vi "Main.vi"() -> ()   [LabVIEW 2019]
uses:
  <vilib>/Platform/TimedLoop/XDataNode/timing_clust.ctl
  <vilib>/Platform/TimedLoop/XDataNode/nitl_modes.ctl
  <vilib>/Platform/TimedLoop/XDataNode/wakeup.ctl
  <vilib>/myRIO/Instrument Drivers/Onboard IO/DIO/typedefs/DIO Reference.ctl
  <vilib>/myRIO/Common/Instrument Driver Framework/Utilities/typedefs/myRIO Generic Hardware Reference.ctl
  <vilib>/myRIO/Common/Instrument Driver Framework/Utilities/typedefs/Hardware Version Enum.ctl
  <vilib>/myRIO/Common/Instrument Driver Framework/Utilities/typedefs/myRIO v1.0 Reference.ctl
  <vilib>/myRIO/Common/Instrument Driver Framework/Utilities/typedefs/Generic FPGA Reference.ctl
  <vilib>/myRIO/Common/Instrument Driver Framework/myRIO v1.0/DIO/typedefs/DIO Channels List.ctl
  <vilib>/myRIO/Common/Instrument Driver Framework/myRIO v1.0/DIO/typedefs/DIO Channels Enum.ctl
  <vilib>/userDefined/High Color/nirio_resource_hc.ctl
  <vilib>/myRIO/Instrument Drivers/Onboard Devices/Accelerometer/typedefs/Accelerometer Reference.ctl
  <vilib>/myRIO/Common/Instrument Driver Framework/myRIO v1.0/Accelerometer/typedefs/Accelerometer Channels List.ctl
  <vilib>/myRIO/Common/Instrument Driver Framework/myRIO v1.0/Accelerometer/typedefs/Accelerometer Channels Enum.ctl
  <vilib>/myRIO/Common/Instrument Driver Framework/Utilities/vis/Is FPGA Ref Available.vi
  <vilib>/myRIO/Common/Instrument Driver Framework/myRIO v1.0/DIO/vis/myRIO v1.1 Open DIO.vi
  <vilib>/myRIO/Instrument Drivers/Onboard IO/DIO/vis/Read.vi
  <vilib>/myRIO/Common/Instrument Driver Framework/myRIO v1.0/Accelerometer/vis/myRIO v1.1 Open Accelerometer.vi
  <vilib>/myRIO/Instrument Drivers/Onboard Devices/Accelerometer/vis/Read.vi
  <vilib>/myRIO/Instrument Drivers/Onboard IO/DIO/vis/Write.vi
  <vilib>/myRIO/Common/Instrument Driver Framework/Utilities/vis/Validate Channels.vi
  <vilib>/myRIO/Common/Instrument Driver Framework/myRIO v1.0/DIO/vis/myRIO v1.0 Reserve DIO.vi
  <vilib>/myRIO/Common/Instrument Driver Framework/myRIO v1.0/Accelerometer/vis/myRIO v1.0 Reserve Accelerometer.vi
  <vilib>/myRIO/Common/Instrument Driver Framework/myRIO v1.0/Resource Manager/vis/myRIO v1.0 Reserve Channel List.vi
  <vilib>/myRIO/Common/Instrument Driver Framework/myRIO v1.0/DIO/vis/myRIO v1.0 Build MUX Configuration DIO.vi
  <vilib>/myRIO/Common/Instrument Driver Framework/myRIO v1.0/Accelerometer/vis/myRIO v1.0 Build MUX Configuration Accelerometer.vi
  <vilib>/myRIO/Common/Instrument Driver Framework/myRIO v1.0/Resource Manager/vis/myRIO v1.0 Reserve Channel.vi
  <vilib>/myRIO/Common/Instrument Driver Framework/myRIO v1.0/Resource Manager/vis/myRIO v1.0 Unreserve Channel.vi
  <vilib>/myRIO/Common/Instrument Driver Framework/myRIO v1.0/Resource Manager/vis/myRIO v1.0 Create Configuration List.vi
  <vilib>/myRIO/Common/Instrument Driver Framework/myRIO v1.0/Resource Manager/vis/myRIO v1.0 Build Mutex Name.vi
  <vilib>/Utility/VariantDataType/GetNumericInfo.vi
  <vilib>/Utility/error.llb/Error Cluster From Error Code.vi
  <vilib>/myRIO/Common/Instrument Driver Framework/myRIO v1.0/myRIO v1.1 Open.vi
  <vilib>/myRIO/Common/Instrument Driver Framework/Utilities/vis/IO Manager.vi
  <vilib>/myRIO/Common/Instrument Driver Framework/Utilities/vis/Configuration Manager.vi
  <vilib>/myRIO/Common/Instrument Driver Framework/myRIO v1.0/Resource Manager/vis/myRIO v1.0 Configure IO.vi
  <vilib>/myRIO/Common/Instrument Driver Framework/myRIO v1.0/myRIO v1.0 Close.vi
  <vilib>/myRIO/Common/Instrument Driver Framework/myRIO v1.0/DIO/vis/myRIO v1.0 Read DIO.vi
  <vilib>/myRIO/Common/Instrument Driver Framework/myRIO v1.0/Accelerometer/vis/myRIO v1.0 Get Scaling Constant Accelerometer.vi
  <vilib>/myRIO/Common/Instrument Driver Framework/myRIO v1.0/Accelerometer/vis/myRIO v1.0 Read Accelerometer.vi
  <vilib>/myRIO/Common/Instrument Driver Framework/myRIO v1.0/DIO/vis/myRIO v1.0 Write DIO.vi
  <vilib>/platform/TimedLoop/XDataNode/XDataNode.xnode
  <vilib>/myRIO/Express VI/Onboard Devices/Button/Button Express VI.xnode
  <vilib>/myRIO/Instrument Drivers/Onboard IO/DIO/vis/myRIO DIO Open.xnode
  <vilib>/myRIO/Express VI/Onboard Devices/Accelerometer/Accelerometer Express VI.xnode
  <vilib>/myRIO/Instrument Drivers/Onboard Devices/Accelerometer/vis/myRIO Accelerometer Open.xnode
  <vilib>/myRIO/Express VI/Onboard Devices/LED/LED Express VI.xnode
  <vilib>/Platform/TimedLoop/XDataNode/XDNodeRunTimeDep.lvlib
  <vilib>/myRIO/Instrument Drivers/Onboard IO/DIO/DIO.lvlib
  <vilib>/myRIO/Instrument Drivers/Onboard Devices/Accelerometer/Accelerometer.lvlib
panel:
  out "error out":errorcluster
  out "AngleTable":dbl[](array[numeric])
  in  "error in (no error)":errorcluster
  out "Axis":dbl[][](array[numeric])
  in  "stop 2":bool
  in  "stop":bool
  # "Angle par défaut du niveau"
  # "Axe en temps réel"
  # "Le s"
  # "Bouton stop en variable partagée semble être une meilleure solution ( impossible à tester concretement sans myRIO )"
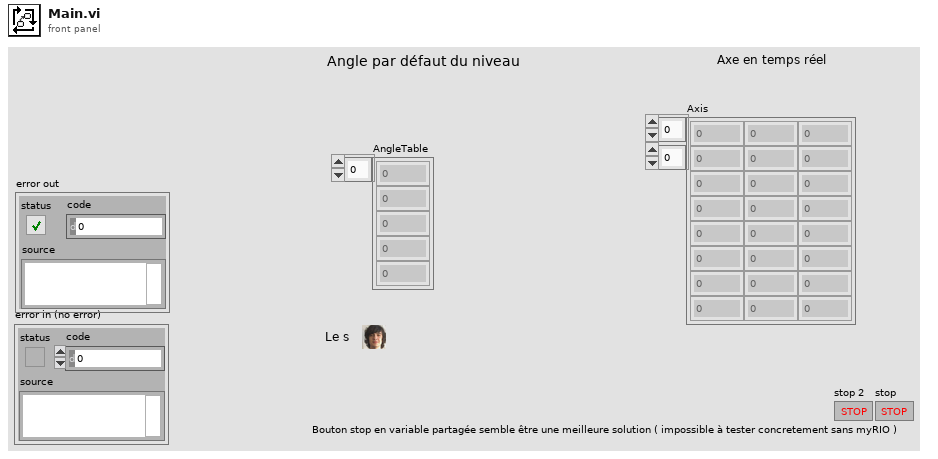
[diagram p1: front panel]
types:
  T1 = enum16{"open", "replace", "create", "open or create", "replace or create", "replace or create with confirmation"}
  T2 = typedef "DIO.lvlib/DIO Reference.ctl" = cluster{"myRIO Reference":T3, "DIO Channels List":T7}
  T3 = typedef "myRIO Generic Hardware Reference.ctl" = cluster{"myRIO Model":T4, "myRIO Hardware Reference":T5}
  T4 = typedef "Hardware Version Enum.ctl" = enum16{"Unknown", "myRIO-1900", "myRIO-1950", "roboRIO", "NI ELVIS RIO CM", "ELVIS III"}
  T5 = typedef "myRIO v1.0 Reference.ctl" = cluster{"Generic FPGA Reference":T6, "Allow multiple opens":bool}
  T6 = typedef "Generic FPGA Reference.ctl" = refnum<k20>
  T7 = typedef "DIO Channels List.ctl" = T8[]
  T8 = typedef "DIO Channels Enum.ctl" = enum16{"Not Connected", "C/DIO0", "C/DIO1", "C/DIO2", "C/DIO3", "C/DIO4", "C/DIO5", "C/DIO6", "C/DIO7", "A/DIO0", "A/DIO1", "A/DIO2", "A/DIO3", "A/DIO4", "A/DIO5", "A/DIO6", "A/DIO7", "A/DIO8", "A/DIO9", "A/DIO10", "A/DIO11", "A/DIO12", "A/DIO13", "A/DIO14", "A/DIO15", "A/DIO16", "A/DIO17", "A/DIO18", "A/DIO19", "B/DIO0", "B/DIO1", "B/DIO2", "B/DIO3", "B/DIO4", "B/DIO5", "B/DIO6", "B/DIO7", "B/DIO8", "B/DIO9", "B/DIO10", "B/DIO11", "B/DIO12", "B/DIO13", "B/DIO14", "B/DIO15", "B/DIO16", "B/DIO17", "B/DIO18", "B/DIO19", "LED0", "LED1", "LED2", "LED3", "Button0", "DIO/DIO0", "DIO/DIO1", "DIO/DIO2", "DIO/DIO3", "DIO/DIO4", "DIO/DIO5", "DIO/DIO6", "DIO/DIO7", "DIO/DIO8", "DIO/DIO9", "SPI/CS0", "SPI/CS1", "SPI/CS2", "SPI/CS3", "LED RADIO (Green)", "LED RADIO (Red)", "LED COMM (Green)", "LED COMM (Red)", "LED MODE (Green)", "LED MODE (Red)"}
  T9 = typedef "nirio_resource_hc.ctl" = tag
  T10 = typedef "Accelerometer.lvlib/Accelerometer Reference.ctl" = cluster{"myRIO Reference":T3, "Accelerometer Channels List":T11, "LSB Weight":dbl}
  T11 = typedef "Accelerometer Channels List.ctl" = T12[]
  T12 = typedef "Accelerometer Channels Enum.ctl" = enum16{"Not Connected", "X-Axis", "Y-Axis", "Z-Axis"}
  T13 = typedef "XDNodeRunTimeDep.lvlib/timing_clust.ctl" = cluster{"Expected End [f-1]":u64, "Actual End [f-1]":u64, "Finished Late? [f-1]":bool, "Expected End [i-1]":u64, "Actual End [i-1]":u64, "Finished Late? [i-1]":bool, "Expected Start [i]":u64, "Actual Start [i]":u64, "Expected Start [f]":u64, "Actual Start [f]":u64, "Source Name":string, "Structure Name":string, "Period":i64, "Deadline":i64, "Offset":i64, "Start":i64, "Priority":i32, "Timeout":i32, "Mode":T14, "Wakeup Reason":T15, "Error":errorcluster, "Source Type":string, "Secondary Source Type":string, "Global End Time":u64, "Global Start Time":u64, "Frame Duration":u64, "Iteration Duration":u64, "Assigned CPU":i32, "I/O Scan Engine Mode":u32}
  T14 = typedef "XDNodeRunTimeDep.lvlib/nitl_modes.ctl" = enum32{"No Change", "Process missed periods, maintain original phase", "Discard missed periods, maintain original phase", "Process missed periods, ignore original phase", "Discard missed periods, ignore original phase"}
  T15 = typedef "XDNodeRunTimeDep.lvlib/wakeup.ctl" = enum32{"Normal", "Aborted", "Asynchronous wakeup", "Timing source error", "Timed loop error", "Timeout"}
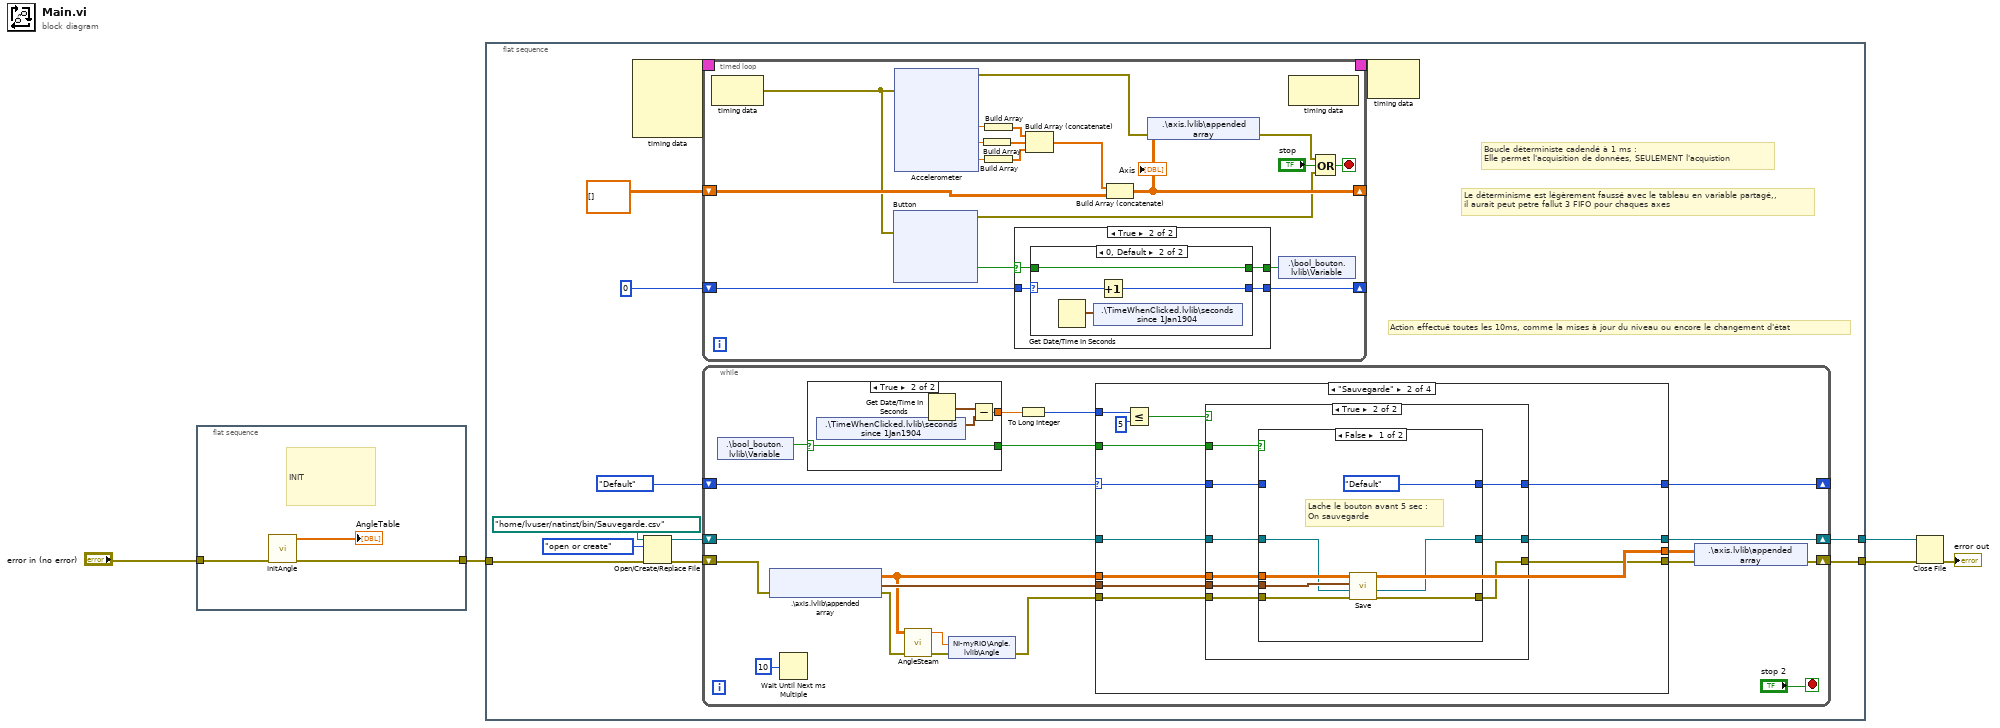
[diagram p0: block diagram]
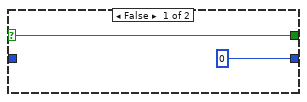
[diagram p2: hidden frame]
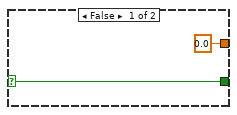
[diagram p4: hidden frame]
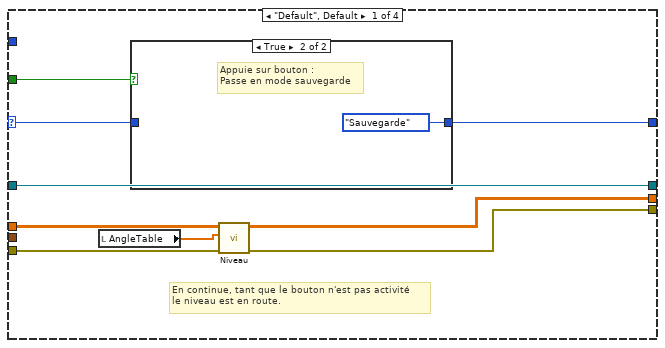
[diagram p5: hidden frame]
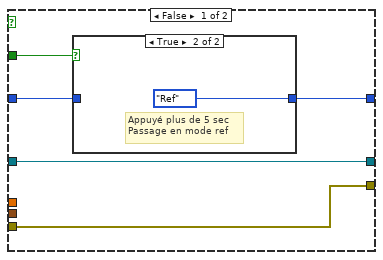
[diagram p7: hidden frame]
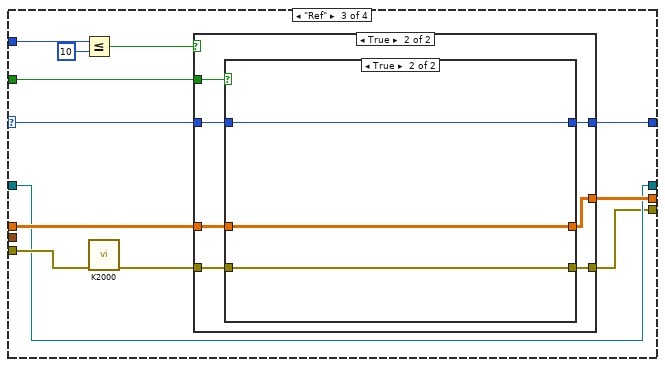
[diagram p10: hidden frame]
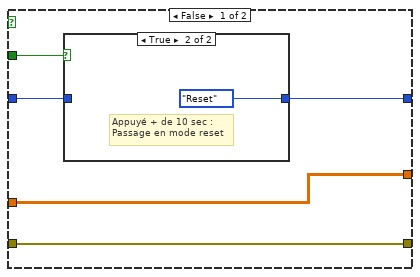
[diagram p11: hidden frame]
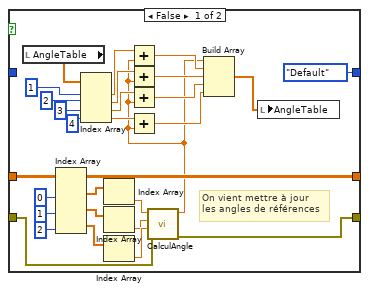
[diagram p13: hidden frame]
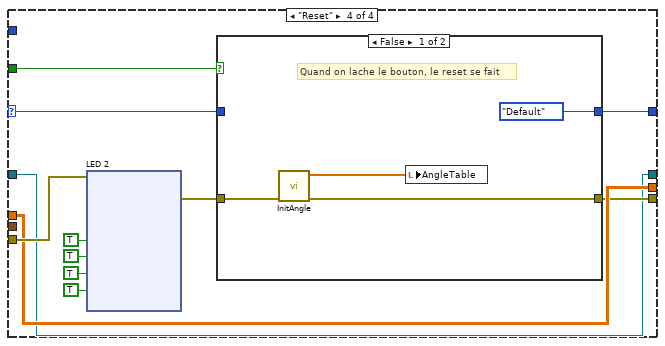
[diagram p14: hidden frame]
diagram:
  n1 = flat-sequence {
    tunnel: "error in (no error)" -> [w8]
    tunnel: [w7] -> w4
    frame #0 {
      # "INIT"
      n2 = call "InitAngle.vi"("error in (no error)"=w8) -> ("error out"=w7:errorcluster, "AngleTable"=→"AngleTable":dbl[])  [unwired: 9 in]
    }
  }
  n3 = flat-sequence {
    tunnel: w4 -> [w12]
    tunnel: [w11] -> w3
    tunnel: [w10] -> w2
    frame #0 {
      # "Action effectué toutes les 10ms, comme la mises à jour du niveau ou encore le changement d'état"
      # "Le déterminisme est légèrement faussé avec le tableau en variable partagé,,\nil aurait peut petre fallut 3 FIFO pour chaques axes"
      # "Boucle déterministe cadendé à 1 ms :\nElle permet l'acquisition de données, SEULEMENT l'acquistion"
      n4 = node-c288() -> (w20:T13)  [unwired: 4 in]
      n5 = Open/Create/Replace File(file path (use dialog)=path "/home/lvuser/natinst/bin/Sauvegarde.csv", error in=w12, operation (0:open)=T1."open or create") -> (refnum out=w9:refnum<file>, error out=w13:errorcluster)  [unwired: 3 in, 1 out]
      n6 = timed-loop {
        timing: w20 -> [_]
        timing-out: [_] -> w19
        shift-right: [w32] -> _
        shift-left: dbl[][] [] -> [w33]
        shift-right: [w28] -> _
        shift-left: 0 -> [w29]
        stop <- w23 stop-if-true
        n7 = node-c288() -> (w27:errorcluster)  [unwired: 1 in]
        n8 = xnode "Button"("error in (no error)"=w27) -> ("Value"=w30:bool, "error out"=w24:errorcluster)
        n9 = xnode "Accelerometer"("error in (no error)"=w27) -> ("Xaxis"=w21:dbl, "Yaxis"=w38:dbl, "Zaxis"=w39:dbl, "error out"=w31:errorcluster)
        n10 = Build Array(w38) -> (w36:dbl[])
        n11 = Build Array(w21) -> (w35:dbl[])
        n12 = Build Array(w39) -> (w37:dbl[])
        n13 = case shown="True" w30 {
          selector: w30 -> [w40 w43]
          tunnel: w29 -> [_ w45]
          tunnel: [0 w44] -> w28
          tunnel: [w40 w42] -> w22
          frame False {
          }
          frame True {
            n14 = case shown="0, Default" w45 {
              selector: w45 -> [w47 w51]
              tunnel: [w47 w50] -> w44
              tunnel: [w46 w49] -> w42
              tunnel: w43 -> [w46 w49]
              frame 1 {
              }
              frame 0, Default {
                n15 = Get Date/Time In Seconds() -> (seconds since 1Jan1904=w48:timestamp)
                n16 = shared-variable ".\\TimeWhenClicked.lvlib\\seconds since 1Jan1904"(w48) -> ()  [unwired: 1 in, 1 out]
                n17 = Increment(x=w51) -> (x+1=w50:i32)
              }
            }
          }
        }
        n18 = Build Array (concatenate)(w35, w36, w37) -> (w34:dbl[])
        n19 = Build Array (concatenate)(w34, w33) -> (w32:dbl[][])
        "Axis" <- w32
        n20 = shared-variable ".\\axis.lvlib\\appended array"(w32, error in=w31) -> (error out=w26:errorcluster)
        n21 = shared-variable ".\\bool_bouton.lvlib\\Variable"(w22) -> ()  [unwired: 1 in, 1 out]
        n22 = node-c288() -> ()  [unwired: 1 in, 1 out]
        n23 = Compound Arithmetic op=OR(w26, "stop", w24) -> (w23:bool)
      }
      n24 = while {
        shift-right: [w144] -> _
        shift-left: enum16{"Default", "Sauvegarde", "Ref", "Reset"}."Default" -> [w147]
        shift-right: [w148] -> w11
        shift-left: w13 -> [w137]
        shift-right: [w143] -> w10
        shift-left: w9 -> [w141]
        stop <- "stop 2" stop-if-true
        n25 = shared-variable ".\\bool_bouton.lvlib\\Variable"() -> (w136:bool)  [unwired: 1 in, 1 out]
        n26 = shared-variable ".\\axis.lvlib\\appended array"(error in=w137) -> (w135:dbl[][], error out=w134:errorcluster, w142:timestamp)
        n27 = Wait Until Next ms Multiple(millisecond multiple=u32 10) -> ()  [unwired: 1 out]
        n28 = case shown="True" w136 {
          selector: w136 -> [w152 w156]
          tunnel: [w152 w156] -> w139
          tunnel: [0.0 w153] -> w138
          frame False {
          }
          frame True {
            n29 = shared-variable ".\\TimeWhenClicked.lvlib\\seconds since 1Jan1904"() -> (w154:timestamp)  [unwired: 1 in, 1 out]
            n30 = Get Date/Time In Seconds() -> (seconds since 1Jan1904=w155:timestamp)
            n31 = Subtract(x=w155, y=w154) -> (x-y=w153:dbl)
          }
        }
        n32 = call "AngleSteam.vi"("error in"=w134, "appended array"=w135) -> ("error out"=w132:errorcluster, "Angle"=w133:dbl)  [unwired: 8 in]
        n33 = shared-variable "NI-myRIO\\Angle.lvlib\\Angle"(w133, error in=w132) -> (error out=w131:errorcluster)
        n34 = To Long Integer(number=w138) -> (32bit integer=w140:i32)
        n35 = case shown="\"Sauvegarde\"" w147 {
          selector: w147 -> [w159 w176 w212 w267]
          tunnel: w135 -> [w165 w173 w210 w266]
          tunnel: w131 -> [w164 w171 w211 w270]
          tunnel: [w163 w173 w209 w266] -> w146
          tunnel: [w162 w172 w206 w264] -> w145
          tunnel: w139 -> [w161 w174 w213 w269]
          tunnel: [w160 w177 w214 w268] -> w144
          tunnel: w140 -> [_ w179 w216 _]
          tunnel: [w157 w170 w208 w263] -> w143
          tunnel: w142 -> [_ w169 _ _]
          tunnel: w141 -> [w157 w168 w208 w263]
          frame "Default", Default {
            # "En continue, tant que le bouton n'est pas activité\nle niveau est en route."
            n36 = local read "AngleTable"() -> (w158:dbl[])
            n37 = case shown="True" w161 {
              tunnel: [w166 enum16{"Default", "Sauvegarde", "Ref", "Reset"}."Sauvegarde"] -> w160
              tunnel: w159 -> [w166 _]
              frame False {
              }
              frame True {
                # "Appuie sur bouton :\nPasse en mode sauvegarde"
              }
            }
            n38 = call "Niveau.vi"("error in (no error)"=w164, "AngleTable"=w158, "Axis entrant"=w165) -> ("error out"=w162:errorcluster, "Axis sortant"=w163:dbl[][])  [unwired: 7 in]
          }
          frame "Sauvegarde" {
            n39 = Less Or Equal?(x=w179, y=5) -> (x <= y?=w175:bool)
            n40 = case shown="True" w175 {
              tunnel: [w184 w194] -> w177
              tunnel: w176 -> [w183 w193]
              tunnel: w174 -> [w182 w195]
              tunnel: w173 -> [_ w192]
              tunnel: w171 -> [w181 w191]
              tunnel: [w181 w190] -> w172
              tunnel: [w180 w189] -> w170
              tunnel: w169 -> [_ w188]
              tunnel: w168 -> [w180 w187]
              frame False {
                n41 = case shown="True" w182 {
                  tunnel: [w185 enum16{"Default", "Sauvegarde", "Ref", "Reset"}."Ref"] -> w184
                  tunnel: w183 -> [w185 _]
                  frame False {
                  }
                  frame True {
                    # "Appuyé plus de 5 sec \nPassage en mode ref"
                  }
                }
              }
              frame True {
                n42 = case shown="False" w195 {
                  tunnel: [enum16{"Default", "Sauvegarde", "Ref", "Reset"}."Default" w205] -> w194
                  tunnel: w193 -> [_ w205]
                  tunnel: w192 -> [w201 _]
                  tunnel: w191 -> [w200 w204]
                  tunnel: [w199 w204] -> w190
                  tunnel: [w198 w203] -> w189
                  tunnel: w188 -> [w197 _]
                  tunnel: w187 -> [w196 w203]
                  frame False {
                    # "Lache le bouton avant 5 sec :\nOn sauvegarde"
                    n43 = call "Save.vi"("error in (no error)"=w200, "refnum in"=w196, "time stamp"=w197, "array"=w201) -> ("error out"=w199:errorcluster, "refnum out"=w198:refnum<file>)  [unwired: 6 in]
                  }
                  frame True {
                  }
                }
              }
            }
          }
          frame "Ref" {
            n44 = Less Or Equal?(x=w216, y=10) -> (x <= y?=w215:bool)
            n45 = call "K2000.vi"("error constant"=w211) -> ("error constant 2"=w207:errorcluster)  [unwired: 10 in]
            n46 = case shown="True" w215 {
              tunnel: [w222 w230] -> w214
              tunnel: w213 -> [w219 w231]
              tunnel: w212 -> [w218 w229]
              tunnel: w210 -> [w221 w228]
              tunnel: [w221 w227] -> w209
              tunnel: w207 -> [w220 w226]
              tunnel: [w220 w225] -> w206
              frame False {
                n47 = case shown="True" w219 {
                  tunnel: [w223 enum16{"Default", "Sauvegarde", "Ref", "Reset"}."Reset"] -> w222
                  tunnel: w218 -> [w223 _]
                  frame False {
                  }
                  frame True {
                    # "Appuyé + de 10 sec :\nPassage en mode reset"
                  }
                }
              }
              frame True {
                n48 = case shown="True" w231 {
                  tunnel: [enum16{"Default", "Sauvegarde", "Ref", "Reset"}."Default" w262] -> w230
                  tunnel: w229 -> [_ w262]
                  tunnel: w228 -> [w258 w261]
                  tunnel: [w258 w261] -> w227
                  tunnel: w226 -> [w233 w260]
                  tunnel: [w232 w260] -> w225
                  frame False {
                    # "On vient mettre à jour\nles angles de références"
                    n49 = local read "AngleTable"() -> (w257:dbl[])
                    n50 = Index Array(array=w258, index (col) #1=0 ("disabled index (col)"), index (col) #2=1 ("index (col)"), index (col) #3=2 ("index (col)")) -> (element #1=w240:dbl[], element #2=w235:dbl[], element #3=w237:dbl[])  [unwired: 3 in]
                    n51 = Index Array(array=w257, index #1=1 ("index"), index #2=2 ("index"), index #3=3 ("index"), index #4=4 ("index")) -> (element #1=w252:dbl, element #2=w251:dbl, element #3=w250:dbl, element #4=w249:dbl)
                    n52 = Index Array(array=w240) -> (element=w239:dbl)  [unwired: 1 in]
                    n53 = Index Array(array=w235) -> (element=w234:dbl)  [unwired: 1 in]
                    n54 = Index Array(array=w237) -> (element=w236:dbl)  [unwired: 1 in]
                    n55 = call "CalculAngle.vi"("error constant"=w233, "Zaxis"=w236, "Yaxis"=w234, "Xaxis"=w239) -> ("error constant 2"=w232:errorcluster, "Numeric"=w238:dbl)  [unwired: 6 in]
                    n56 = Add(x=w252, y=w238) -> (x+y=w248:dbl)
                    n57 = Add(x=w251, y=w238) -> (x+y=w247:dbl)
                    n58 = Add(x=w250, y=w238) -> (x+y=w245:dbl)
                    n59 = Add(x=w249, y=w238) -> (x+y=w246:dbl)
                    n60 = Build Array(w238, w248, w247, w245, w246) -> (w244:dbl[])
                    n61 = local write "AngleTable"(w244) -> ()
                  }
                  frame True {
                  }
                }
              }
            }
          }
          frame "Reset" {
            n62 = xnode "LED 2"("L0"=TRUE, "L1"=TRUE ("L0"), "L2"=TRUE ("L0"), "L3"=TRUE ("L0"), "error in (no error)"=w270) -> ("error out"=w265:errorcluster)
            n63 = case shown="False" w269 {
              tunnel: [enum16{"Default", "Sauvegarde", "Ref", "Reset"}."Default" w280] -> w268
              tunnel: w267 -> [_ w280]
              tunnel: w265 -> [w277 w279]
              tunnel: [w276 w279] -> w264
              frame False {
                # "Quand on lache le bouton, le reset se fait"
                n64 = call "InitAngle.vi"("error in (no error)"=w277) -> ("error out"=w276:errorcluster, "AngleTable"=w275:dbl[])  [unwired: 9 in]
                n65 = local write "AngleTable"(w275) -> ()
              }
              frame True {
              }
            }
          }
        }
        n66 = shared-variable ".\\axis.lvlib\\appended array"(w146, error in=w145) -> (error out=w148:errorcluster)
      }
      n67 = node-c288(w19) -> ()  [unwired: 1 out]
    }
  }
  n68 = Close File(refnum=w2, error in=w3) -> (error out=→"error out":errorcluster)  [unwired: 1 out]
